vi "Robot Global Data.vi"() -> ()   [LabVIEW 2014]
doc: "This global VI can contain as many global variables as you need. Place a control on the panel, give it a good name. To read or write to it from a VI, drag the icon to the diagram of that VI. You can also drag from the project. Click on the node to change which global you access. You shouldn't have multiple locations writing to a global or it will cause a race-condition."
uses:
  <vilib>/Rock Robotics/WPI/Camera/WPI_CameraImageSize.ctl
  <vilib>/Rock Robotics/WPI/DriverStation/WPI_DriverStationRobotMode2.ctl
panel:
  in  "NEW CODE":bool
  out "Burgler_OUTPUT":bool
  out "Burgler":bool
  out "Btn_SuckStop":bool
  in  "PID":bool
  out "AUTO":bool
  out "Temp":dbl
  out "North":dbl
  out "Header":dbl
  in  "PID gains":T1={"proportional gain (Kc)"=0.021, "integral time (Ti, min)"=0.0, "derivative time (Td, min)"=0.0} {"derivative time (Td, min)" format="%.3f"; "integral time (Ti, min)" format="%.3f"; "proportional gain (Kc)" format="%.3f"}
  out "Btn_SuckOut":bool
  out "Btn_SuckIn":bool
  out "Btn_ManualForksOff":bool
  out "Btn_ManualForksOn":bool
  out "Forks BtnOutput":bool
  out "Manual Forklift BtnOutput":bool
  out "Manual StackFunction":bool
  out "Btn_ManualDriveToggle":bool
  out "Brake Out?":bool
  out "Right Switch":bool
  out "Left Switch":bool
  out "Manual Forklift":bool
  out "At Level?":bool
  out "Btn_HPS_InitialSet":bool
  out "HPS_FirstTote?":bool
  out "Btn_HPS":bool
  out "ForksStop":bool
  out "BackDrive":bool
  out "Btn_StrafeRight":bool
  out "Btn_StrafeLeft":bool
  out "Wanted Level":dbl
  out "Current Level":dbl
  out "Btn_StackFunction":bool
  out "Btn_ForkliftDown":bool
  out "Btn_ForkliftUp":bool
  out "Btn_Forks":bool
  out "NAVX_Heading":dbl
  in  "Torque Release":bool
  in  "Robot Mode":T2
  in  "image size":T3=enum."320x240"
  in  "Enable Vision":bool
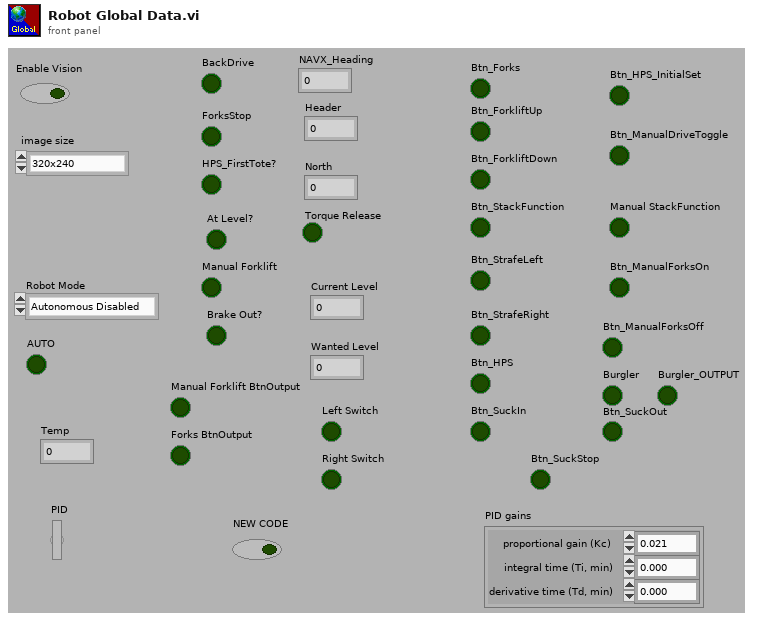
[diagram p1: front panel]
types:
  T1 = cluster{"proportional gain (Kc)":dbl, "integral time (Ti, min)":dbl, "derivative time (Td, min)":dbl}
  T2 = typedef "WPI_DriverStationRobotMode2.ctl" = enum16{"Autonomous Disabled", "Autonomous Enabled", "Teleop Disabled", "Teleop Enabled", "Disconnected", "Finish", "Test Disabled", "Test Enabled", "Emergency Stopped"}
  T3 = typedef "WPI_CameraImageSize.ctl" = enum16{"640x480", "320x240", "160x120", "Custom"}
diagram:
